vi "AssertControlValueNotEqual.vi"(0 "VI Reference In":refnum<vi>, 1 "Label":string, 5 "Control Name":string, 7 "Control Value":variant, 9 "Timeout(5 sec)":dbl=5.0, 11 "Error In":errorcluster, 12 "Assert Interval(10 ms)":u32=10) -> (4 "VI Reference Out":refnum<vi>, 15 "Error Out":errorcluster)   [LabVIEW 2016]
doc: "<b>This VI asserts if the value of controls is not equal to the given value in other VI.<b> \n\nThe input control name is given as a string , incase of path, use delimiters inbetween the path.\nThis VI gets the value of the control, untill the value is not equal to the input value."
uses:
  AssertControlValueByPathString.vi
  <vilib>/addons/_JKI Toolkits/Caraya/classes/Assert/Assert Not Equal Value and Type_Variant.vi
  <vilib>/addons/_JKI Toolkits/Caraya/classes/Assert/Assert.lvclass
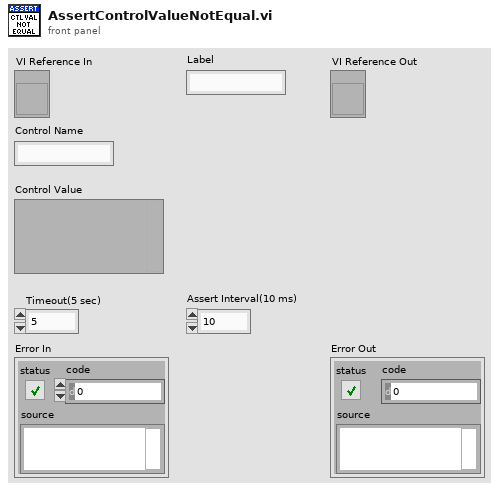
[diagram p1: front panel]
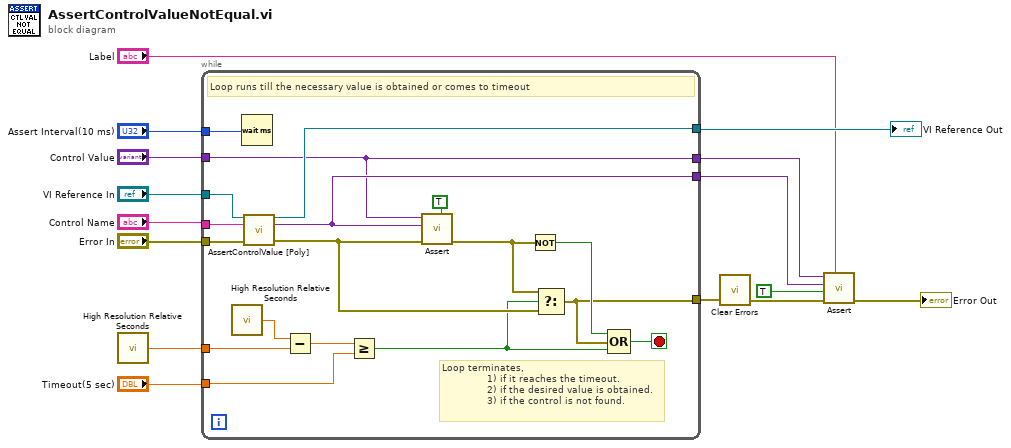
[diagram p0: block diagram]
diagram:
  n1 = call <vilib>:"High Resolution Relative Seconds.vi"() -> ("relative seconds"=w12:dbl)
  n2 = while {
    tunnel: "Control Name" -> [w32]
    tunnel: "VI Reference In" -> [w31]
    tunnel: "Control Value" -> [w21]
    tunnel: "Timeout(5 sec)" -> [w26]
    tunnel: [w28] -> w9
    tunnel: w12 -> [w30]
    tunnel: "Error In" -> [w33]
    tunnel: [w18] -> w2
    tunnel: [w21] -> w7
    tunnel: [w22] -> w6
    tunnel: "Assert Interval(10 ms)" -> [w16]
    stop <- w24 stop-if-true
    # "Loop terminates,\n               1) if it reaches the timeout.\n               2) if the desired value is obtained.\n               3) if the control is not found."
    # "Loop runs till the necessary value is obtained or comes to timeout"
    n3 = call <vilib>:"High Resolution Relative Seconds.vi"() -> ("relative seconds"=w29:dbl)
    n4 = Wait (ms)(milliseconds to wait=w16) -> ()  [unwired: 1 out]
    n5 = call-poly "AssertControlValue [Poly].vi"("VI Reference In"=w31, "Control Name"=w32, "error in"=w33) -> ("VI Reference Out"=w28:refnum<vi>, "Value"=w22:variant, "error out"=w25:errorcluster)  [unwired: 10 in]
    n6 = Subtract(x=w29, y=w30) -> (x-y=w27:dbl)
    n7 = Greater Or Equal?(x=w27, y=w26) -> (x >= y?=w20:bool)
    n8 = call-poly <vilib>:"Assert.vi"("Assert Only? (F)"=TRUE, "error in (no error)"=w25, "Y"=w22, "X"=w21) -> ("error out"=w23:errorcluster)  [unwired: 7 in]
    n9 = Not(x=w23) -> (.not. x?=w19:bool)
    n10 = Select(t=w23, s=w20, f=w25) -> (s? t:f=w18:errorcluster)
    n11 = Compound Arithmetic op=OR(w19, w18, w20) -> (w24:bool)
  }
  "VI Reference Out" <- w9
  n12 = call <vilib>:"Clear Errors.vi"("error in (no error)"=w2) -> ("error out"=w8:errorcluster)  [unwired: 5 in, 1 out]
  n13 = call-poly <vilib>:"Assert.vi"("Label"="Label", "error in (no error)"=w8, "Register with caller test (F)"=TRUE, "Y"=w6, "X"=w7) -> ("error out"=→"Error Out":errorcluster)  [unwired: 6 in]
